vi "DialogLoop.vi"(8 "Error In":errorcluster, 11 "Message Queues":T1) -> (0 "Error Out":errorcluster)   [LabVIEW 2017, in "Server.lvlib" / "Dialogs.lvlib"]
uses:
  Dialogs.lvlib
  Message Queue/CommReferences.ctl
  Message Queue/MessageCluster.ctl
  DialogLoopData.ctl
  TypeDefs/ServerINI.ctl
  Oracle/OracleData.ctl
  <vilib>/Utility/error.llb/Error Cluster From Error Code.vi
  <vilib>/ErrorRing/Error Ring.xnode
  Message Queue/Message Queue.lvlib
  ErrorLogger/ErrorLogger.lvlib
  Oracle/Oracle.lvlib
  Server.lvlib
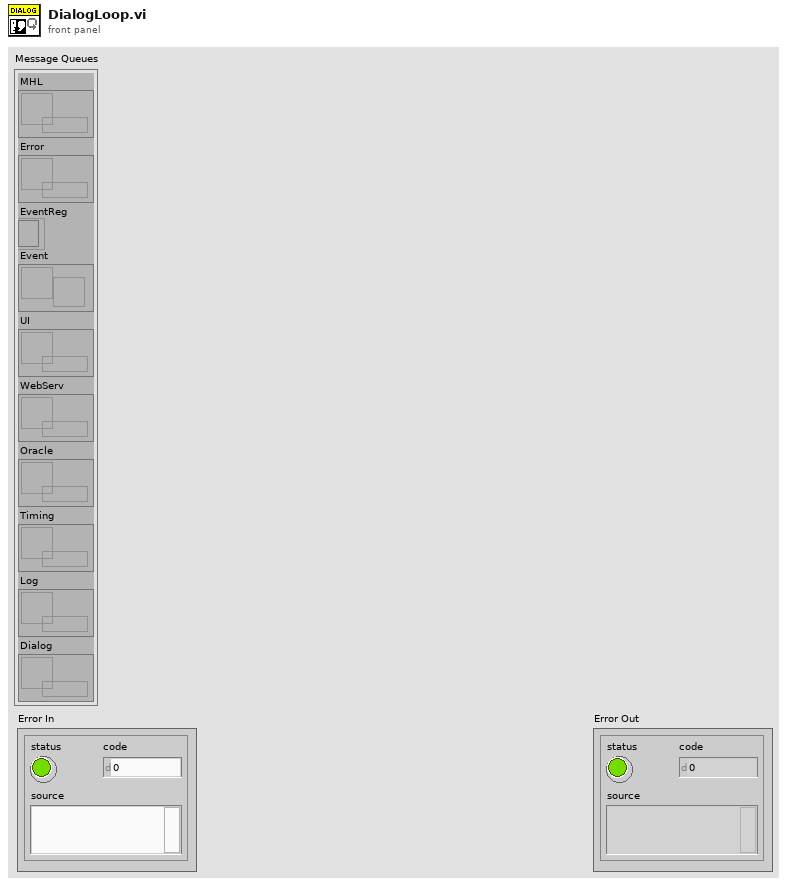
[diagram p1: front panel]
types:
  T1 = typedef "Server.lvlib/Message Queue.lvlib/CommReferences.ctl" = cluster{"MHL":refnum<queue>, "Error":refnum<queue>, "EventReg":refnum<event-registration>, "Event":refnum<user-event>, "UI":refnum<queue>, "WebServ":refnum<queue>, "Oracle":refnum<queue>, "Timing":refnum<queue>, "Log":refnum<queue>, "Dialog":refnum<queue>}
  T2 = typedef "Server.lvlib/Dialogs.lvlib/DialogLoopData.ctl" = cluster{"ServerINI":T3}
  T3 = typedef "Server.lvlib/ServerINI.ctl" = cluster{"TrackQueues?":bool, "ClientTimeout (s)":u32, "LogPath":path, "ErrorsToIgnore":i32[], "OracleData":T4}
  T4 = typedef "Server.lvlib/Oracle.lvlib/OracleData.ctl" = cluster{"DBname":string, "User":string, "Password":string}
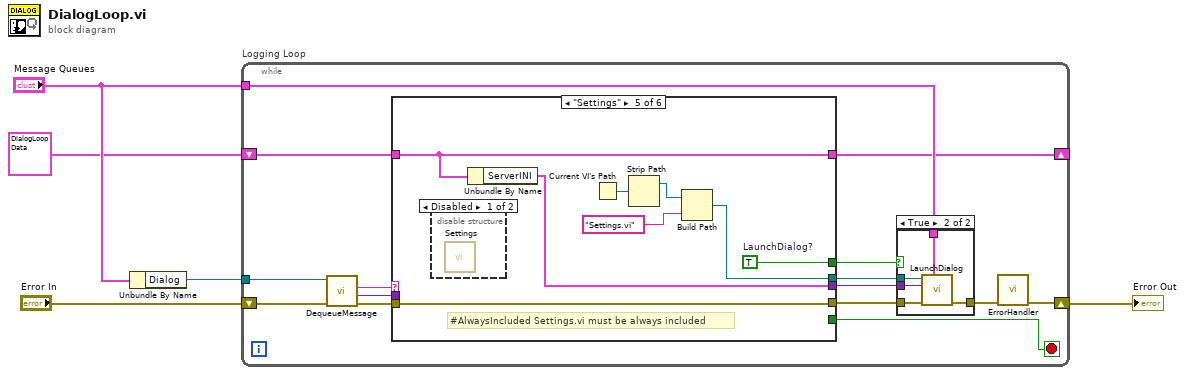
[diagram p0: block diagram]
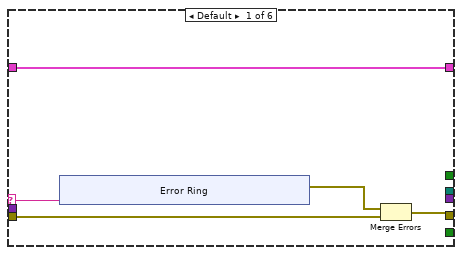
[diagram p3: hidden frame]
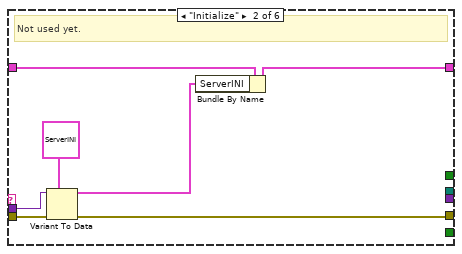
[diagram p4: hidden frame]
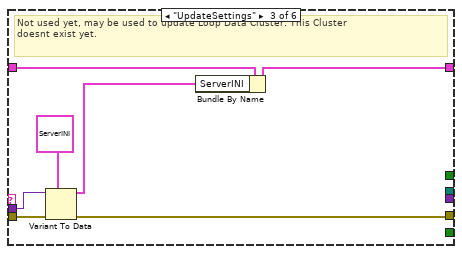
[diagram p5: hidden frame]
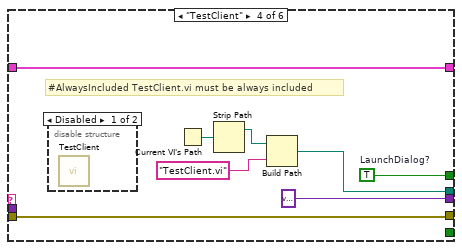
[diagram p6: hidden frame]
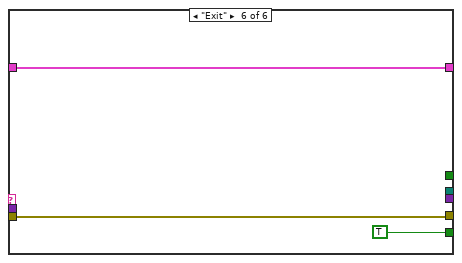
[diagram p9: hidden frame]
diagram:
  n1 = Unbundle By Name("Message Queues") -> ("Dialog"=w5:refnum<queue>)
  n2 = while "Logging Loop" {
    shift-right: [w14] -> w4
    shift-left: "Error In" -> [w20]
    tunnel: w5 -> [w19]
    tunnel: "Message Queues" -> [w9]
    shift-right: [w6] -> _
    shift-left: T2 {"ServerINI"={"TrackQueues?"=TRUE, "ClientTimeout (s)"=30, "LogPath"=path "C:/Users/jgoebel/Documents/GitHub/AEDashboard/ServerLib/Data/ServerLog.tdms", "ErrorsToIgnore"=[], "OracleData"={"DBname"="", "User"="", "Password"=""}}} ("DialogLoopData") -> [w7]
    stop <- w15 stop-if-true
    n3 = call "DequeueMessage.vi"("error in (no error)"=w20, "Message Queue"=w19) -> ("error out"=w18:errorcluster, "Message Data"=w16:variant, "Message"=w13:string)  [unwired: 5 in, 2 out]
    n4 = case shown="\"Settings\"" w13 {
      selector: w13 -> [w30 _ _ _ _ _]
      tunnel: [w29 w44 w49 w60 w68 w71] -> w17
      tunnel: w18 -> [w31 w45 w52 w60 w68 w71]
      tunnel: w16 -> [_ w43 w48 _ _ _]
      tunnel: [_ _ _ _ _ TRUE] -> w15
      tunnel: [_ _ _ w54 w63 _] -> w11
      tunnel: [_ _ _ w59 w67 _] -> w10
      tunnel: [_ _ _ variant w61 _] -> w8
      tunnel: [w27 w40 w50 w53 w62 w69] -> w6
      tunnel: w7 -> [w27 w41 w51 w53 w62 w69]
      frame Default {
        n5 = xnode "Error Ring"("parameter 0"=w30) -> ("error out"=w28:errorcluster)
        n6 = Merge Errors(w28, w31) -> (w29:errorcluster)
      }
      frame "Initialize" {
        # "Not used yet."
        n7 = Variant To Data(error in=w45, type=T3 {"TrackQueues?"=TRUE, "ClientTimeout (s)"=30, "LogPath"=path "C:/Users/jgoebel/Documents/GitHub/AEDashboard/ServerLib/Data/ServerLog.tdms", "ErrorsToIgnore"=[], "OracleData"={"DBname"="", "User"="", "Password"=""}} ("ServerINI"), Variant=w43) -> (data=w39:T3, error out=w44:errorcluster)
        n8 = Bundle By Name(cluster=w41, "ServerINI"=w39) -> (w40:T2)
      }
      frame "UpdateSettings" {
        # "Not used yet, may be used to update Loop Data Cluster. This Cluster\ndoesnt exist yet."
        n9 = Variant To Data(error in=w52, type=T3 {"TrackQueues?"=TRUE, "ClientTimeout (s)"=30, "LogPath"=path "C:/Users/jgoebel/Documents/GitHub/AEDashboard/ServerLib/Data/ServerLog.tdms", "ErrorsToIgnore"=[], "OracleData"={"DBname"="", "User"="", "Password"=""}} ("ServerINI"), Variant=w48) -> (data=w46:T3, error out=w49:errorcluster)
        n10 = Bundle By Name(cluster=w51, "ServerINI"=w46) -> (w50:T2)
      }
      frame "TestClient" {
        w59 = TRUE  # LaunchDialog?
        # "#AlwaysIncluded TestClient.vi must be always included"
        n11 = disable-structure shown="Disabled" {
          frame Disabled {
            n12 = call "TestClient.vi"() -> ()  [unwired: 12 in]
          }
          frame Enabled {
          }
        }
        n13 = Current VI's Path() -> (path=w57:path)
        n14 = Strip Path(path=w57) -> (stripped path=w56:path)  [unwired: 1 out]
        n15 = Build Path(base path=w56, name or relative path="TestClient.vi") -> (appended path=w54:path)
      }
      frame "Settings" {
        w67 = TRUE  # LaunchDialog?
        # "#AlwaysIncluded Settings.vi must be always included"
        n16 = disable-structure shown="Disabled" {
          frame Disabled {
            n17 = call "Settings.vi"() -> ()  [unwired: 12 in]
          }
          frame Enabled {
          }
        }
        n18 = Unbundle By Name(w62) -> ("ServerINI"=w61:T3)
        n19 = Current VI's Path() -> (path=w66:path)
        n20 = Strip Path(path=w66) -> (stripped path=w65:path)  [unwired: 1 out]
        n21 = Build Path(base path=w65, name or relative path="Settings.vi") -> (appended path=w63:path)
      }
      frame "Exit" {
      }
    }
    n22 = case shown="True" w10 {
      tunnel: w17 -> [w21 w26]
      tunnel: [w21 w25] -> w12
      tunnel: w11 -> [_ w24]
      tunnel: w9 -> [_ w23]
      tunnel: w8 -> [_ w22]
      frame False {
      }
      frame True {
        n23 = call "LaunchDialog.vi"("Queues"=w23, "error in (no error)"=w26, "DialogData"=w22, "DialogPath"=w24) -> ("error out"=w25:errorcluster)  [unwired: 7 in]
      }
    }
    n24 = call "ErrorHandler.vi"("error in (no error)"=w12) -> ("error out"=w14:errorcluster)  [unwired: 10 in]
  }
  "Error Out" <- w4
